vi "configureAnalogOutput.vi"(8 "error in (no error)":errorcluster, 9 "AnalogOutput":refnum<class "AnalogOutput.lvclass">, 10 "deviceName":string, 11 "BECHWCBasic in":refnum<class "BECHWCBasic.lvclass">) -> (0 "error out":errorcluster, 3 "BECHWCBasic out":refnum<class "BECHWCBasic.lvclass">)   [LabVIEW 2011, in "Hardware.lvlib" / "HWControllers.lvlib" / "BECHWCBasic.lvclass"]
doc: "Configure the analog channels of a device"
uses:
  BECHWCBasic.lvclass
  Channels/VoltOutput/AnalogOutput.lvclass
  BECHWCBasic.lvclass/BECHWCBasic.ctl
  HWController.lvclass
  Tools/Filing/FileNeologist/FileNeologist.lvclass
  Tools/Filing.lvlib
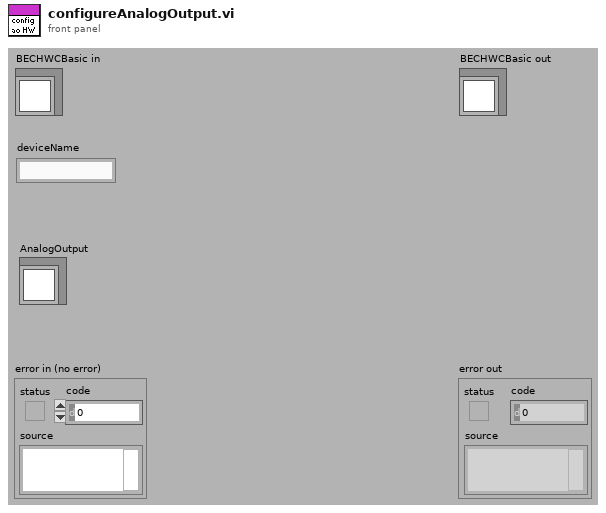
[diagram p1: front panel]
types:
  T1 = cluster{string, "Physical Channels":string, "Ranges":dbl[]}
  T2 = cluster{"Clock source":string, "Clock rate":dbl, "Start trigger line":string, "Sample Rate":dbl, "Sample No.":dbl}
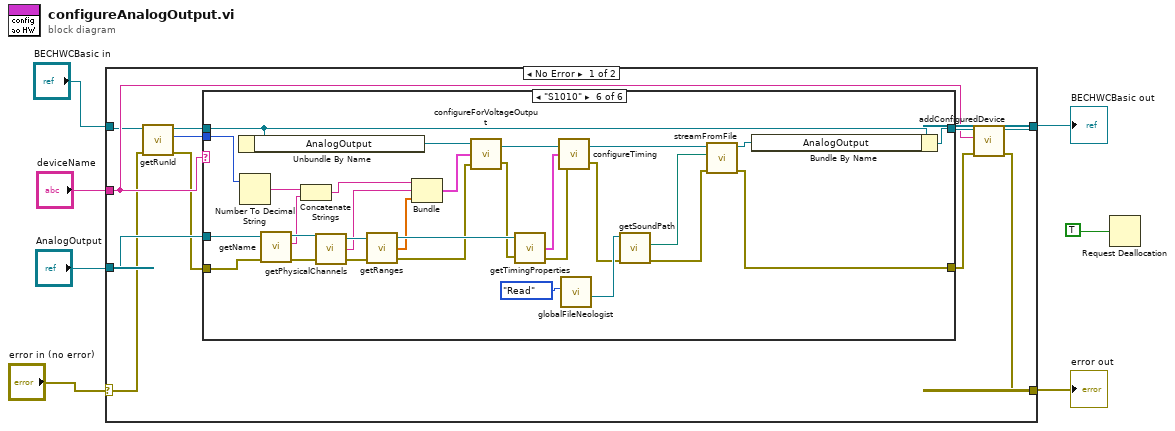
[diagram p0: block diagram]
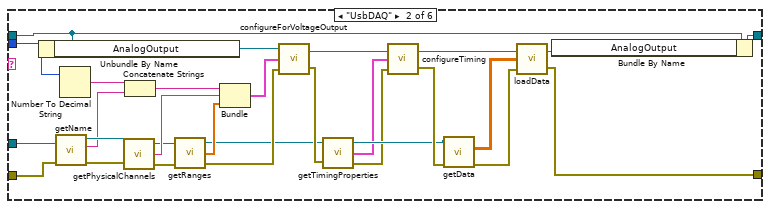
[diagram p3: hidden frame]
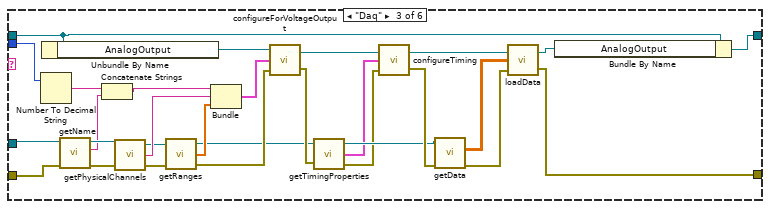
[diagram p4: hidden frame]
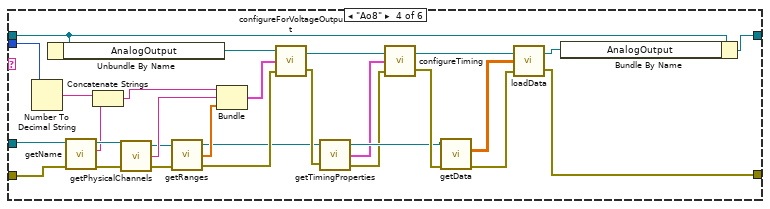
[diagram p5: hidden frame]
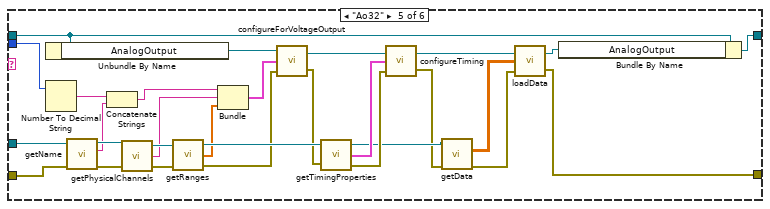
[diagram p6: hidden frame]
diagram:
  n1 = case shown="No Error" "error in (no error)" {
    selector: "error in (no error)" -> [w10 w168]
    tunnel: [w14 w168] -> w6
    tunnel: [w16 w167] -> w4
    tunnel: "BECHWCBasic in" -> [w11 w167]
    tunnel: "deviceName" -> [w13 _]
    tunnel: "AnalogOutput" -> [w18 _]
    frame No Error {
      n2 = call "getRunId.vi"("error in (no error)"=w10, "HWController in"=w11) -> ("error out"=w9:errorcluster, "Numeric"=w8:i32, "HWController out"=w12:refnum<class "BECHWCBasic.lvclass">)  [unwired: 7 in]
      n3 = case shown="\"S1010\"" w13 {
        tunnel: w12 -> [w20 w29 w58 w87 w136 w166]
        tunnel: [w20 w28 w57 w86 w135 w165] -> w17
        tunnel: [w19 w27 w56 w85 w112 w143] -> w15
        tunnel: w18 -> [_ w26 w55 w84 w128 w158]
        tunnel: w9 -> [w19 w25 w54 w83 w129 w159]
        tunnel: w8 -> [_ w21 w52 w81 w110 w147]
        frame "No Hardware", Default {
        }
        frame "UsbDAQ" {
          n4 = Unbundle By Name(w29) -> ("AnalogOutput"=w35:refnum<class "AnalogOutput.lvclass">)
          n5 = call "getName.vi"("error in (no error)"=w25, "AnalogOutput.lvclass in"=w26) -> ("error out"=w30:errorcluster, "name"=w23:string, "AnalogOutput.lvclass out"=w32:refnum<class "AnalogOutput.lvclass">)  [unwired: 7 in]
          n6 = Number To Decimal String(number=w21) -> (decimal integer string=w24:string)  [unwired: 1 in]
          n7 = call-dynamic "getPhysicalChannels.vi"("AnalogOutput.lvclass in"=w32, "error in (no error)"=w30) -> ("AnalogOutput.lvclass out"=w33:refnum<class "AnalogOutput.lvclass">, "Physical Channels"=w36:string, "error out"=w31:errorcluster)
          n8 = Concatenate Strings(w24, w23) -> (w22:string)
          n9 = call "getRanges.vi"("AnalogOutput.lvclass in"=w33, "error in (no error)"=w31) -> ("AnalogOutput.lvclass out"=w34:refnum<class "AnalogOutput.lvclass">, "Ranges"=w37:dbl[], "error out"=w39:errorcluster)
          n10 = Bundle(w22, "Physical Channels"=w36, "Ranges"=w37) -> (w38:T1)  [unwired: 1 in]
          n11 = call-dynamic "configureForVoltageOutput.vi"("error in (no error)"=w39, "Output Properties"=w38, "AnalogOutput in"=w35) -> ("error out"=w40:errorcluster, "AnalogOutput out"=w44:refnum<class "AnalogOutput.lvclass">)
          n12 = call "getTimingProperties.vi"("AnalogOutput.lvclass in"=w34, "error in (no error)"=w40) -> ("AnalogOutput.lvclass out"=w43:refnum<class "AnalogOutput.lvclass">, "Timing"=w42:T2, "error out"=w41:errorcluster)
          n13 = call-dynamic "configureTiming.vi"("error in (no error)"=w41, "Timing"=w42, "AnalogOutput in"=w44) -> ("error out"=w48:errorcluster, "AnalogOutput out"=w45:refnum<class "AnalogOutput.lvclass">)
          n14 = call "getData.vi"("error in (no error)"=w48, "AnalogOutput.lvclass in"=w43) -> ("error out"=w47:errorcluster, "Data"=w46:dbl[][])  [unwired: 7 in, 1 out]
          n15 = call-dynamic "loadData.vi"("error in (no error)"=w47, "Data"=w46, "AnalogOutput in"=w45) -> ("error out"=w27:errorcluster, "AnalogOutput out"=w49:refnum<class "AnalogOutput.lvclass">)
          n16 = Bundle By Name(cluster=w29, "AnalogOutput"=w49) -> (w28:refnum<class "BECHWCBasic.lvclass">)
        }
        frame "Daq" {
          n17 = Number To Decimal String(number=w52) -> (decimal integer string=w53:string)  [unwired: 1 in]
          n18 = Unbundle By Name(w58) -> ("AnalogOutput"=w64:refnum<class "AnalogOutput.lvclass">)
          n19 = call "getName.vi"("error in (no error)"=w54, "AnalogOutput.lvclass in"=w55) -> ("error out"=w59:errorcluster, "name"=w51:string, "AnalogOutput.lvclass out"=w61:refnum<class "AnalogOutput.lvclass">)  [unwired: 7 in]
          n20 = Concatenate Strings(w53, w51) -> (w50:string)
          n21 = call-dynamic "getPhysicalChannels.vi"("AnalogOutput.lvclass in"=w61, "error in (no error)"=w59) -> ("AnalogOutput.lvclass out"=w62:refnum<class "AnalogOutput.lvclass">, "Physical Channels"=w65:string, "error out"=w60:errorcluster)
          n22 = call "getRanges.vi"("AnalogOutput.lvclass in"=w62, "error in (no error)"=w60) -> ("AnalogOutput.lvclass out"=w63:refnum<class "AnalogOutput.lvclass">, "Ranges"=w66:dbl[], "error out"=w68:errorcluster)
          n23 = Bundle(w50, "Physical Channels"=w65, "Ranges"=w66) -> (w67:T1)  [unwired: 1 in]
          n24 = call-dynamic "configureForVoltageOutput.vi"("error in (no error)"=w68, "Output Properties"=w67, "AnalogOutput in"=w64) -> ("error out"=w69:errorcluster, "AnalogOutput out"=w73:refnum<class "AnalogOutput.lvclass">)
          n25 = call "getTimingProperties.vi"("AnalogOutput.lvclass in"=w63, "error in (no error)"=w69) -> ("AnalogOutput.lvclass out"=w72:refnum<class "AnalogOutput.lvclass">, "Timing"=w71:T2, "error out"=w70:errorcluster)
          n26 = call-dynamic "configureTiming.vi"("error in (no error)"=w70, "Timing"=w71, "AnalogOutput in"=w73) -> ("error out"=w77:errorcluster, "AnalogOutput out"=w74:refnum<class "AnalogOutput.lvclass">)
          n27 = call "getData.vi"("error in (no error)"=w77, "AnalogOutput.lvclass in"=w72) -> ("error out"=w76:errorcluster, "Data"=w75:dbl[][])  [unwired: 7 in, 1 out]
          n28 = call-dynamic "loadData.vi"("error in (no error)"=w76, "Data"=w75, "AnalogOutput in"=w74) -> ("error out"=w56:errorcluster, "AnalogOutput out"=w78:refnum<class "AnalogOutput.lvclass">)
          n29 = Bundle By Name(cluster=w58, "AnalogOutput"=w78) -> (w57:refnum<class "BECHWCBasic.lvclass">)
        }
        frame "Ao8" {
          n30 = Number To Decimal String(number=w81) -> (decimal integer string=w82:string)  [unwired: 1 in]
          n31 = Unbundle By Name(w87) -> ("AnalogOutput"=w93:refnum<class "AnalogOutput.lvclass">)
          n32 = call "getName.vi"("error in (no error)"=w83, "AnalogOutput.lvclass in"=w84) -> ("error out"=w88:errorcluster, "name"=w80:string, "AnalogOutput.lvclass out"=w90:refnum<class "AnalogOutput.lvclass">)  [unwired: 7 in]
          n33 = Concatenate Strings(w82, w80) -> (w79:string)
          n34 = call-dynamic "getPhysicalChannels.vi"("AnalogOutput.lvclass in"=w90, "error in (no error)"=w88) -> ("AnalogOutput.lvclass out"=w91:refnum<class "AnalogOutput.lvclass">, "Physical Channels"=w94:string, "error out"=w89:errorcluster)
          n35 = call "getRanges.vi"("AnalogOutput.lvclass in"=w91, "error in (no error)"=w89) -> ("AnalogOutput.lvclass out"=w92:refnum<class "AnalogOutput.lvclass">, "Ranges"=w95:dbl[], "error out"=w97:errorcluster)
          n36 = Bundle(w79, "Physical Channels"=w94, "Ranges"=w95) -> (w96:T1)  [unwired: 1 in]
          n37 = call-dynamic "configureForVoltageOutput.vi"("error in (no error)"=w97, "Output Properties"=w96, "AnalogOutput in"=w93) -> ("error out"=w98:errorcluster, "AnalogOutput out"=w102:refnum<class "AnalogOutput.lvclass">)
          n38 = call "getTimingProperties.vi"("AnalogOutput.lvclass in"=w92, "error in (no error)"=w98) -> ("AnalogOutput.lvclass out"=w101:refnum<class "AnalogOutput.lvclass">, "Timing"=w100:T2, "error out"=w99:errorcluster)
          n39 = call-dynamic "configureTiming.vi"("error in (no error)"=w99, "Timing"=w100, "AnalogOutput in"=w102) -> ("error out"=w106:errorcluster, "AnalogOutput out"=w103:refnum<class "AnalogOutput.lvclass">)
          n40 = call "getData.vi"("error in (no error)"=w106, "AnalogOutput.lvclass in"=w101) -> ("error out"=w105:errorcluster, "Data"=w104:dbl[][])  [unwired: 7 in, 1 out]
          n41 = call-dynamic "loadData.vi"("error in (no error)"=w105, "Data"=w104, "AnalogOutput in"=w103) -> ("error out"=w85:errorcluster, "AnalogOutput out"=w107:refnum<class "AnalogOutput.lvclass">)
          n42 = Bundle By Name(cluster=w87, "AnalogOutput"=w107) -> (w86:refnum<class "BECHWCBasic.lvclass">)
        }
        frame "Ao32" {
          n43 = Unbundle By Name(w136) -> ("AnalogOutput"=w127:refnum<class "AnalogOutput.lvclass">)
          n44 = Number To Decimal String(number=w110) -> (decimal integer string=w111:string)  [unwired: 1 in]
          n45 = call "getName.vi"("error in (no error)"=w129, "AnalogOutput.lvclass in"=w128) -> ("error out"=w134:errorcluster, "name"=w109:string, "AnalogOutput.lvclass out"=w132:refnum<class "AnalogOutput.lvclass">)  [unwired: 7 in]
          n46 = Concatenate Strings(w111, w109) -> (w108:string)
          n47 = call-dynamic "getPhysicalChannels.vi"("AnalogOutput.lvclass in"=w132, "error in (no error)"=w134) -> ("AnalogOutput.lvclass out"=w131:refnum<class "AnalogOutput.lvclass">, "Physical Channels"=w126:string, "error out"=w133:errorcluster)
          n48 = call "getRanges.vi"("AnalogOutput.lvclass in"=w131, "error in (no error)"=w133) -> ("AnalogOutput.lvclass out"=w130:refnum<class "AnalogOutput.lvclass">, "Ranges"=w125:dbl[], "error out"=w123:errorcluster)
          n49 = Bundle(w108, "Physical Channels"=w126, "Ranges"=w125) -> (w124:T1)  [unwired: 1 in]
          n50 = call-dynamic "configureForVoltageOutput.vi"("error in (no error)"=w123, "Output Properties"=w124, "AnalogOutput in"=w127) -> ("error out"=w122:errorcluster, "AnalogOutput out"=w118:refnum<class "AnalogOutput.lvclass">)
          n51 = call "getTimingProperties.vi"("AnalogOutput.lvclass in"=w130, "error in (no error)"=w122) -> ("AnalogOutput.lvclass out"=w119:refnum<class "AnalogOutput.lvclass">, "Timing"=w120:T2, "error out"=w121:errorcluster)
          n52 = call-dynamic "configureTiming.vi"("error in (no error)"=w121, "Timing"=w120, "AnalogOutput in"=w118) -> ("error out"=w114:errorcluster, "AnalogOutput out"=w117:refnum<class "AnalogOutput.lvclass">)
          n53 = call "getData.vi"("error in (no error)"=w114, "AnalogOutput.lvclass in"=w119) -> ("error out"=w115:errorcluster, "Data"=w116:dbl[][])  [unwired: 7 in, 1 out]
          n54 = call-dynamic "loadData.vi"("error in (no error)"=w115, "Data"=w116, "AnalogOutput in"=w117) -> ("error out"=w112:errorcluster, "AnalogOutput out"=w113:refnum<class "AnalogOutput.lvclass">)
          n55 = Bundle By Name(cluster=w136, "AnalogOutput"=w113) -> (w135:refnum<class "BECHWCBasic.lvclass">)
        }
        frame "S1010" {
          n56 = Unbundle By Name(w166) -> ("AnalogOutput"=w157:refnum<class "AnalogOutput.lvclass">)
          n57 = Number To Decimal String(number=w147) -> (decimal integer string=w148:string)  [unwired: 1 in]
          n58 = call "getName.vi"("error in (no error)"=w159, "AnalogOutput.lvclass in"=w158) -> ("error out"=w164:errorcluster, "name"=w146:string, "AnalogOutput.lvclass out"=w162:refnum<class "AnalogOutput.lvclass">)  [unwired: 7 in]
          n59 = Concatenate Strings(w148, w146) -> (w145:string)
          n60 = call-dynamic "getPhysicalChannels.vi"("AnalogOutput.lvclass in"=w162, "error in (no error)"=w164) -> ("AnalogOutput.lvclass out"=w161:refnum<class "AnalogOutput.lvclass">, "Physical Channels"=w156:string, "error out"=w163:errorcluster)
          n61 = call "getRanges.vi"("AnalogOutput.lvclass in"=w161, "error in (no error)"=w163) -> ("AnalogOutput.lvclass out"=w160:refnum<class "AnalogOutput.lvclass">, "Ranges"=w155:dbl[], "error out"=w153:errorcluster)
          n62 = Bundle(w145, "Physical Channels"=w156, "Ranges"=w155) -> (w154:T1)  [unwired: 1 in]
          n63 = call-dynamic "configureForVoltageOutput.vi"("error in (no error)"=w153, "Output Properties"=w154, "AnalogOutput in"=w157) -> ("error out"=w152:errorcluster, "AnalogOutput out"=w149:refnum<class "AnalogOutput.lvclass">)
          n64 = call "getTimingProperties.vi"("AnalogOutput.lvclass in"=w160, "error in (no error)"=w152) -> ("Timing"=w150:T2, "error out"=w151:errorcluster)  [unwired: 1 out]
          n65 = call-dynamic "configureTiming.vi"("error in (no error)"=w151, "Timing"=w150, "AnalogOutput in"=w149) -> ("error out"=w139:errorcluster, "AnalogOutput out"=w144:refnum<class "AnalogOutput.lvclass">)
          n66 = call "globalFileNeologist.vi"("Action"=enum16{"Write", "Read"}."Read") -> ("FileNeologist out"=w141:refnum<class "FileNeologist.lvclass">)  [unwired: 10 in]
          n67 = call "getSoundPath.vi"("error in (no error)"=w139, "FileNeologist in"=w141) -> ("error out"=w138:errorcluster, "Path"=w137:path)  [unwired: 7 in, 1 out]
          n68 = call-dynamic "streamFromFile.vi"("error in (no error)"=w138, "Path"=w137, "AnalogOutput in"=w144) -> ("error out"=w143:errorcluster, "AnalogOutput out"=w142:refnum<class "AnalogOutput.lvclass">)  [unwired: 7 in]
          n69 = Bundle By Name(cluster=w166, "AnalogOutput"=w142) -> (w165:refnum<class "BECHWCBasic.lvclass">)
        }
      }
      n70 = call "addConfiguredDevice.vi"("error in (no error)"=w15, "deviceName"=w13, "HWController in"=w17) -> ("error out"=w14:errorcluster, "HWController out"=w16:refnum<class "BECHWCBasic.lvclass">)  [unwired: 7 in]
    }
    frame Error {
    }
  }
  "error out" <- w6
  "BECHWCBasic out" <- w4
  n71 = Request Deallocation(TRUE) -> ()
